vi "roi_selection.vi"(6 "Starting Evaluate?":bool, 8 "List Parameter Fit In":dbl[][](array[numeric]), 9 "List ROI In":dbl[][](array[numeric]), 10 "List Peaks":string[][](table), 11 "Spectrum In":cluster{"Locations":dbl[], "Amplitudes":dbl[]}) -> (2 "List Parameter Fit Out":dbl[][](array[numeric]), 3 "List ROI Out":dbl[][](array[numeric]))   [LabVIEW 2023]
uses:
  <vilib>/Analysis/NI_AALPro.lvlib
  <vilib>/Analysis/6fits.llb/Curve Fitting Criteria.ctl
panel:
  out "All Fit Parameters":T1(array[cluster])
  out "Parameters Fit":T2
  out "Fit Values":dbl[][](array[numeric])
  out "standard deviation":dbl
  in  "element":i32
  out "FWHM":dbl
  out "amplitude":dbl
  out "XY Graph 2":cluster{dbl[], "Best Gaussian Fit":dbl[]}[](graph)
  in  "Elements":string[][](table)
  out "XY Graph":cluster{"Channels":dbl[], "Intensity":dbl[]}(graph)
  out "Spectrum":cluster{"Locations":dbl[], "Amplitudes":dbl[]}(graph)
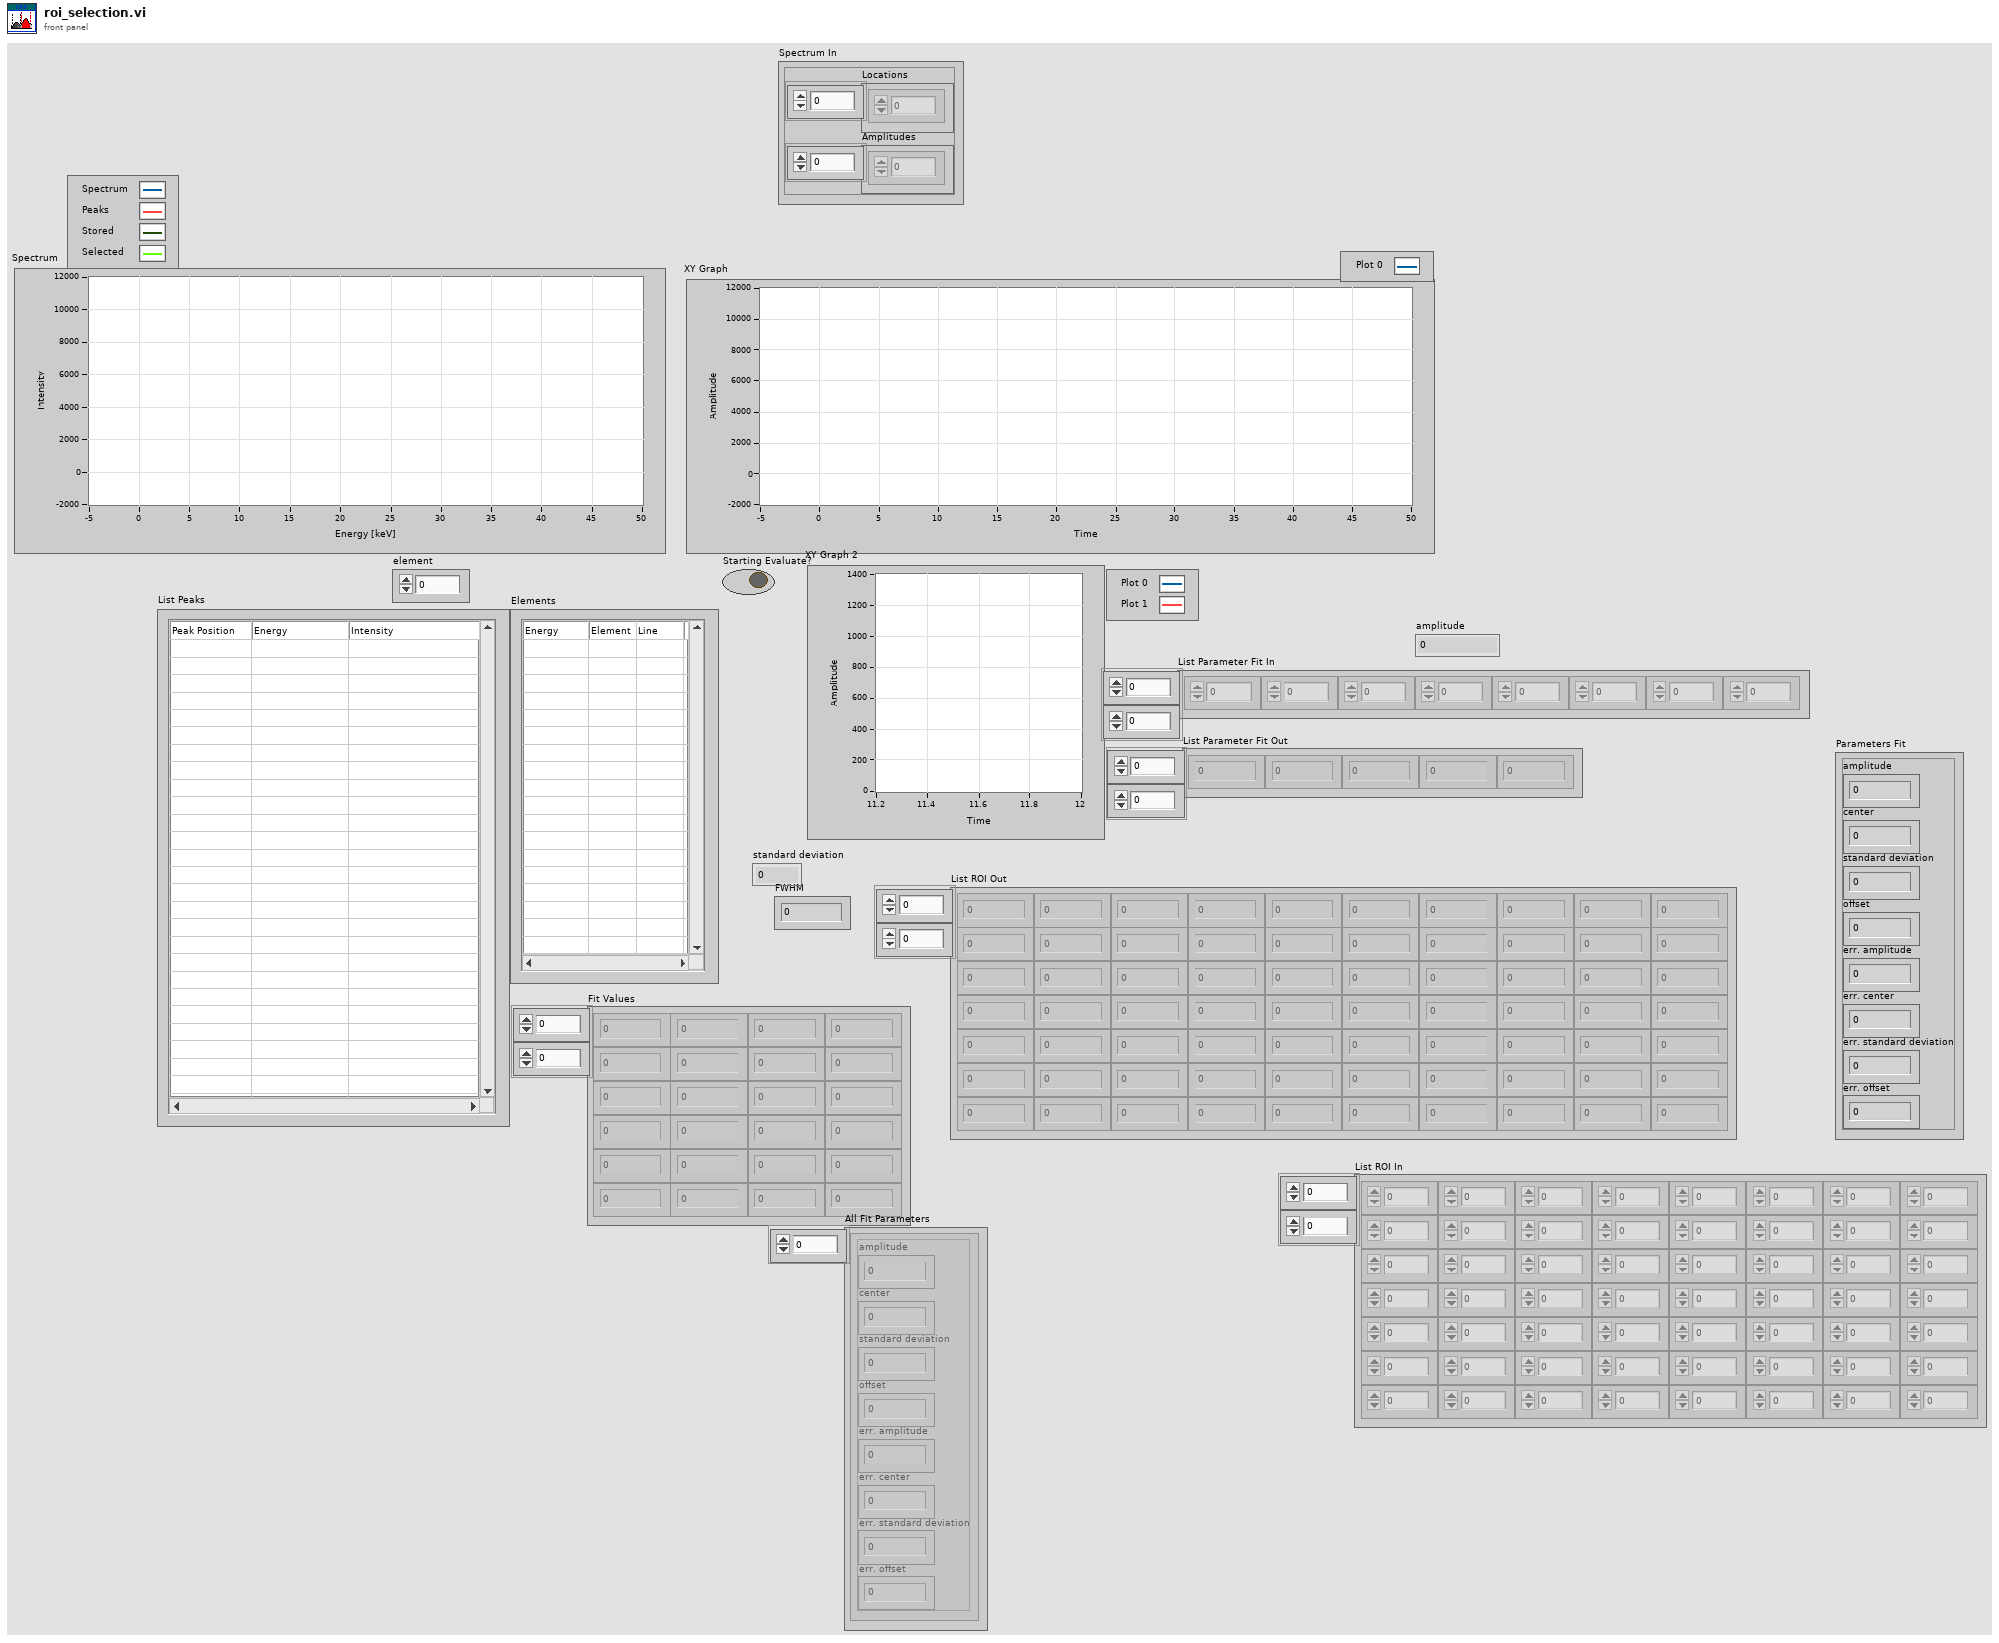
[diagram p1: front panel]
types:
  T1 = cluster{"amplitude":dbl, "center":dbl, "standard deviation":dbl, "offset":dbl, "err. amplitude":dbl, "err. center":dbl, "err. standard deviation":dbl, "err. offset":dbl}[]
  T2 = cluster{"amplitude":dbl, "center":dbl, "standard deviation":dbl, "offset":dbl, "err. amplitude":dbl, "err. center":dbl, "err. standard deviation":dbl, "err. offset":dbl}
  T3 = cluster{"initial amplitude":dbl, "initial center":dbl, "initial standard deviation":dbl, "offset":dbl}
  T4 = typedef "NI_AALPro.lvlib/Curve Fitting Criteria.ctl" = u16
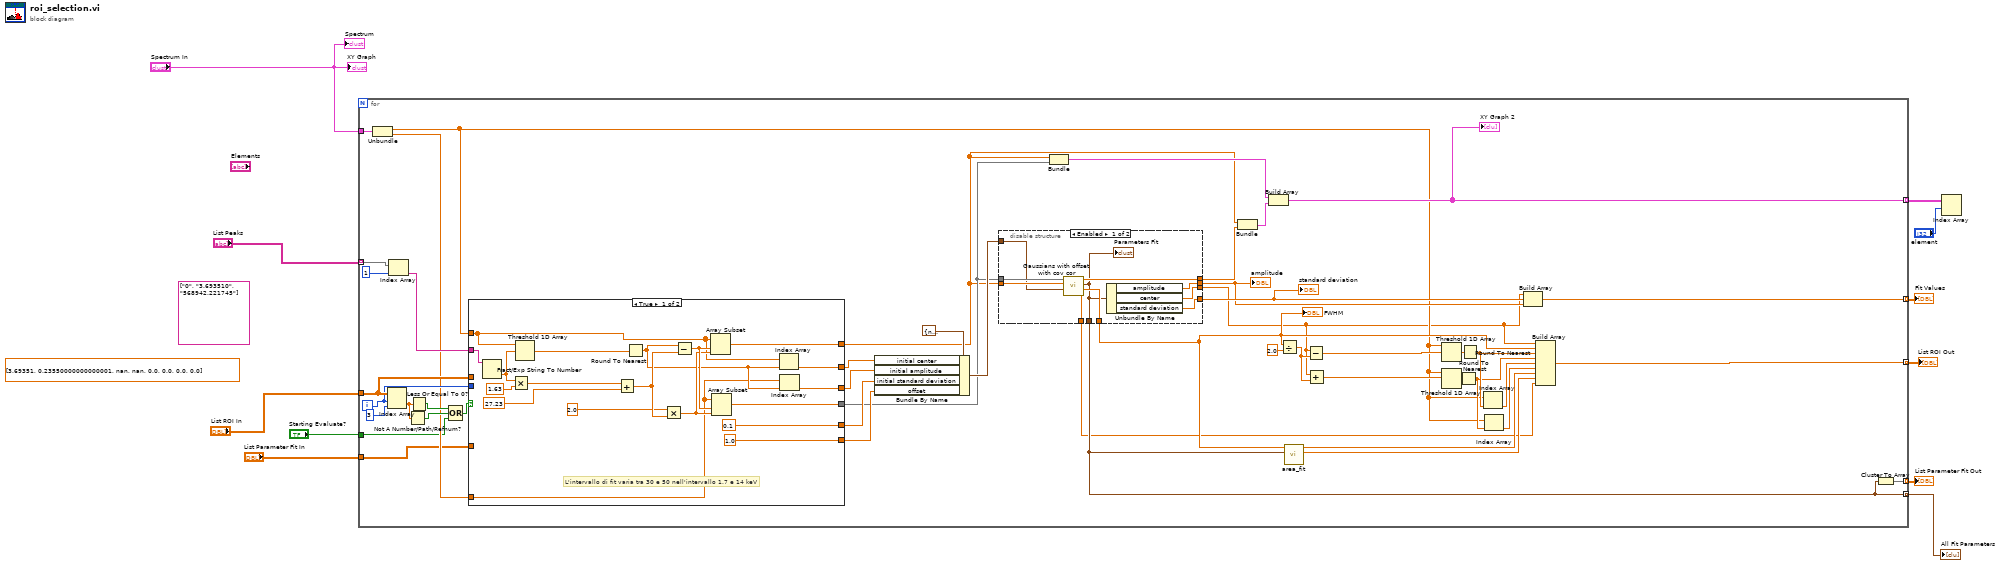
[diagram p0: block diagram]
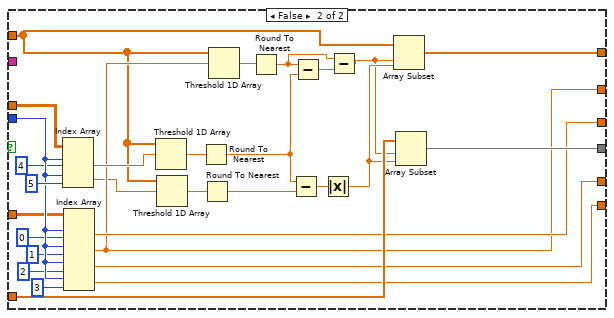
[diagram p2: hidden frame]
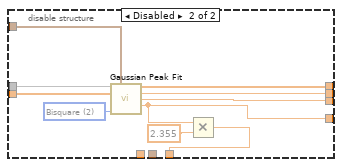
[diagram p3: hidden frame]
diagram:
  (unwired) dbl[][] [[3.69351, 0.23550000000000001, nan, nan, 0.0, 0.0, 0.0, 0.0]] ("List ROI In")
  (unwired) string[][] [["0", "3.693510", "568942.221745"]] ("List Peaks 2")
  n1 = for {
    tunnel: "Spectrum In" -> [w59]
    tunnel: [w49] -> w11 mode=indexing
    tunnel: [w46] -> w9 mode=indexing
    tunnel: "List Peaks" -> [w47] mode=indexing
    tunnel: [w41] -> w7 mode=indexing
    tunnel: [w35] -> w6 mode=indexing
    tunnel: [w34] -> w5 mode=indexing
    tunnel: "List ROI In" -> [w32]
    tunnel: "List Parameter Fit In" -> [w14]
    tunnel: "Starting Evaluate?" -> [w13]
    i -> [w31]
    n2 = Unbundle(w59) -> ("Locations"=w25:dbl[], "Amplitudes"=w24:dbl[])
    n3 = Index Array(array=w32, index (row)=w31, index (col)=3 ("index")) -> (element=w28:dbl)
    n4 = Index Array(array=w47, index=1 ("disabled index (col)")) -> (element=w26:string)
    n5 = Not A Number/Path/Refnum?(number/path/refnum=w28) -> (NaN/Path/Refnum?=w27:bool)
    n6 = Less Or Equal To 0?(x=w28) -> (x <= 0?=w30:bool)
    n7 = Compound Arithmetic op=OR(w30, w27, w13) -> (w29:bool)
    n8 = case shown="True" w29 {
      tunnel: w32 -> [_ w101]
      tunnel: w31 -> [_ w99]
      tunnel: w26 -> [w78 _]
      tunnel: w25 -> [w61 w85]
      tunnel: w24 -> [w60 w104]
      tunnel: [w67 w105] -> w17
      tunnel: [w68 w106] -> w16
      tunnel: [w65 w88] -> w23
      tunnel: [w64 w93] -> w22
      tunnel: [0.1 ("initial standard deviation") w92] -> w19
      tunnel: [1.0 ("offset") w91] -> w18
      tunnel: w14 -> [_ w98]
      frame True {
        # "L'intervallo di fit varia tra 30 e 50 nell'intervallo 1.7 e 14 keV"
        n9 = Fract/Exp String To Number(string=w78) -> (number=w73:dbl)  [unwired: 3 in, 1 out]
        n10 = Multiply(x=w73, y=1.63) -> (x*y=w76:dbl)
        n11 = Threshold 1D Array(2:w73, 3:w61) -> (0:w74:dbl)  [unwired: 1 in]
        n12 = Add(x=w76, y=27.23) -> (x+y=w72:dbl)
        n13 = Round To Nearest(number=w74) -> (nearest integer value=w66:dbl)
        n14 = Multiply(x=2.0, y=w72) -> (x*y=w69:dbl)
        n15 = Subtract(x=w66, y=w72) -> (x-y=w70:dbl)
        n16 = Array Subset(array=w61, index=w70, length=w69) -> (w68:dbl[])
        n17 = Array Subset(array=w60, index=w70, length=w69) -> (w67:dbl[])
        n18 = Index Array(array=w61, index=w66) -> (element=w65:dbl)
        n19 = Index Array(array=w60, index=w66) -> (element=w64:dbl)
      }
      frame False {
        n20 = Index Array(array=w101, index (row) #1=w99, index (col) #1=4 ("disabled index (col)"), index (row) #2=w99, index (col) #2=5 ("disabled index (col)")) -> (element #1=w89:dbl, element #2=w84:dbl)
        n21 = Index Array(array=w98, index (row) #1=w99, index (col) #1=0 ("index (col)"), index (row) #2=w99, index (col) #2=1 ("index (col)"), index (row) #3=w99, index (col) #3=2 ("index (col)"), index (row) #4=w99, index (col) #4=3 ("index (col)")) -> (element #1=w93:dbl, element #2=w88:dbl, element #3=w92:dbl, element #4=w91:dbl)
        n22 = Threshold 1D Array(2:w89, 3:w85) -> (0:w86:dbl)  [unwired: 1 in]
        n23 = Threshold 1D Array(2:w84, 3:w85) -> (0:w87:dbl)  [unwired: 1 in]
        n24 = Round To Nearest(number=w86) -> (nearest integer value=w82:dbl)
        n25 = Round To Nearest(number=w87) -> (nearest integer value=w83:dbl)
        n26 = Threshold 1D Array(2:w88, 3:w85) -> (0:w107:dbl)  [unwired: 1 in]
        n27 = Round To Nearest(number=w107) -> (nearest integer value=w80:dbl)
        n28 = Subtract(x=w82, y=w83) -> (x-y=w103:dbl)
        n29 = Subtract(x=w80, y=w82) -> (x-y=w81:dbl)
        n30 = Absolute Value(x=w103) -> (abs(x)=w100:dbl)
        n31 = Subtract(x=w80, y=w81) -> (x-y=w79:dbl)
        n32 = Array Subset(array=w85, index=w79, length=w100) -> (w106:dbl[])
        n33 = Array Subset(array=w104, index=w79, length=w100) -> (w105:dbl[])
      }
    }
    n34 = Bundle By Name(cluster=T3 {"initial amplitude"=nan, "initial center"=nan, "initial standard deviation"=nan, "offset"=nan} ("initial guess"), "initial center"=w23, "initial amplitude"=w22, "initial standard deviation"=w19, "offset"=w18) -> (w20:T3)
    n35 = disable-structure shown="Enabled" {
      disable-tunnel: w20 -> [w115 w127]
      disable-tunnel: [w114 w126] -> w58
      disable-tunnel: w16 -> [w116 w125]
      disable-tunnel: w17 -> [w117 w124]
      disable-tunnel: [w109 w119] -> w40
      disable-tunnel: [w110 w122] -> w15
      disable-tunnel: [w111 w121] -> w39
      disable-tunnel: [w113 w118] -> w37
      disable-tunnel: [w112 _] -> w35
      disable-tunnel: [w108 _] -> w12
      frame Enabled {
        n36 = call "Gaussians with offset with cov cor.vi"("initial guess"=w115, "X"=w116, "Y"=w117) -> ("R-square"=w108:dbl, "FWHM"=w113:dbl, "Parameters Fit"=w112:T2, "best nonlinear fit"=w114:dbl[])  [unwired: 5 in]
        "Parameters Fit" <- w112
        n37 = Unbundle By Name(w112) -> ("amplitude"=w111:dbl, "center"=w110:dbl, "standard deviation"=w109:dbl)
      }
      frame Disabled {
        w123 = T4 2 items=["Least Square", "Least Absolute Residual", "Bisquare"] ("method")
        n38 = call <vilib>:"Gaussian Peak Fit.vi"("Y"=w124, "initial guess"=w127, "X"=w125, "method"=w123) -> ("Best Gaussian Fit"=w126:dbl[], "amplitude"=w121:dbl, "center"=w122:dbl, "standard deviation"=w119:dbl)  [unwired: 5 in, 3 out]
        n39 = Multiply(x=w119, y=2.355) -> (x*y=w118:dbl)
      }
    }
    "amplitude" <- w39
    "FWHM" <- w37
    "standard deviation" <- w40
    n40 = Bundle(w16, w17) -> (w56:cluster{dbl[], dbl[]})  [unwired: 1 in]
    n41 = Bundle(w16, "best nonlinear fit"=w58) -> (w57:cluster{dbl[], "best nonlinear fit":dbl[]})  [unwired: 1 in]
    n42 = Build Array(w56, w57) -> (w46:cluster{dbl[], "best nonlinear fit":dbl[]}[])
    "XY Graph 2" <- w46
    n43 = Divide(x=w37, y=2.0) -> (x/y=w54:dbl)
    n44 = call "area_fit.vi"("Parameters Fit"=w35, "FWHM"=w37) -> ("Err. Area"=w36:dbl, "Area"=w38:dbl)  [unwired: 8 in]
    n45 = Subtract(x=w15, y=w54) -> (x-y=w52:dbl)
    n46 = Add(x=w15, y=w54) -> (x+y=w53:dbl)
    n47 = Threshold 1D Array(2:w52, 3:w25) -> (0:w51:dbl)  [unwired: 1 in]
    n48 = Threshold 1D Array(2:w53, 3:w25) -> (0:w50:dbl)  [unwired: 1 in]
    n49 = Round To Nearest(number=w50) -> (nearest integer value=w44:dbl)
    n50 = Round To Nearest(number=w51) -> (nearest integer value=w45:dbl)
    n51 = Index Array(array=w25, index=w45) -> (element=w43:dbl)
    n52 = Index Array(array=w25, index=w44) -> (element=w42:dbl)
    n53 = Build Array(w15, w40, w39) -> (w41:dbl[])
    n54 = Build Array(w15, w37, w45, w44, w43, w42, w38, w36, w12) -> (w49:dbl[])
    n55 = Cluster To Array(cluster=w35) -> (array=w34:dbl[])
  }
  "List ROI Out" <- w11
  "Fit Values" <- w7
  "All Fit Parameters" <- w6
  "List Parameter Fit Out" <- w5
  n56 = Index Array(array=w9, index (row)="element") -> ()  [unwired: 1 in, 1 out]
  "Spectrum" <- "Spectrum In"
  "XY Graph" <- "Spectrum In"
